vi "WLAN Configure Signal.vi"(0 "Instrument Handle In":refnum<k21>, 1 "Selector String":string, 5 "WLAN Signal Configuration":T1={"Auto Detect Signal?"=TRUE, "Standard"=0, "Channel Bandwidth (Hz)"=20000000.0} {"Channel Bandwidth (Hz)" items=["5M"=5000000.0, "10M"=10000000.0, "20M"=20000000.0, "40M"=40000000.0, "80M"=80000000.0, "160M"=160000000.0]; "Standard" items=["802.11a/g", "802.11b", "802.11j", "802.11p", "802.11n", "802.11ac", "802.11ax"]}, 11 "error in (no error)":errorcluster) -> (4 "Instrument Handle Out":refnum<k21>, 15 "error out":errorcluster)   [LabVIEW 2016, in "RFmxWLAN.lvlib"]
uses:
  RFmxWLAN.lvlib
  Typedefs/WLAN Signal Configuration.ctl
panel:
  # "OR"
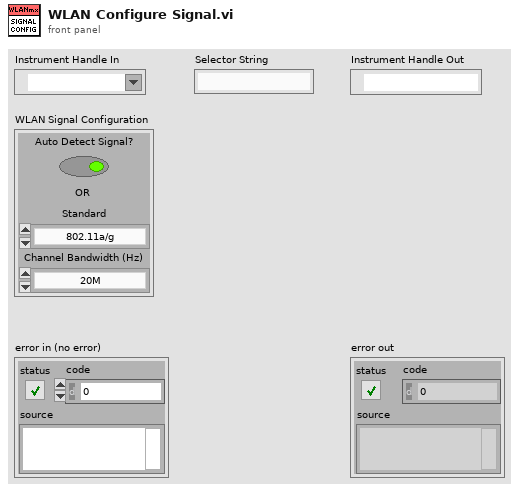
[diagram p1: front panel]
types:
  T1 = typedef "RFmxWLAN.lvlib/WLAN Signal Configuration.ctl" = cluster{"Auto Detect Signal?":bool, "Standard":i32, "Channel Bandwidth (Hz)":dbl}
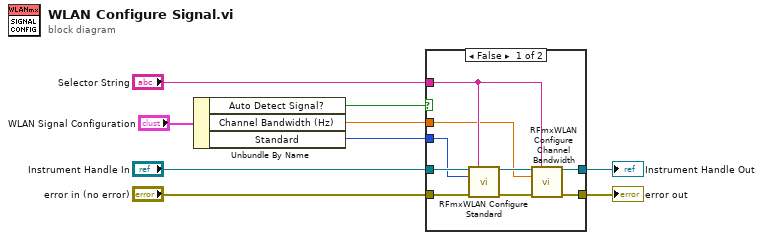
[diagram p0: block diagram]
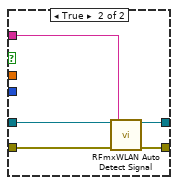
[diagram p2: hidden frame]
diagram:
  n1 = Unbundle By Name("WLAN Signal Configuration") -> ("Auto Detect Signal?"=w3:bool, "Channel Bandwidth (Hz)"=w2:dbl, "Standard"=w1:i32)
  n2 = case shown="False" w3 {
    tunnel: "Instrument Handle In" -> [w18 w23]
    tunnel: "error in (no error)" -> [w17 w22]
    tunnel: [w13 w21] -> w7
    tunnel: [w14 w20] -> w6
    tunnel: "Selector String" -> [w12 w19]
    tunnel: w2 -> [w11 _]
    tunnel: w1 -> [w10 _]
    frame False {
      n3 = call <vilib>:"RFmxWLAN Configure Standard.vi"("Instrument Handle In"=w18, "Selector String"=w12, "Standard"=w10, "error in (no error)"=w17) -> ("Instrument Handle Out"=w16:refnum<k21>, "error out"=w15:errorcluster)  [unwired: 10 in]
      n4 = call <vilib>:"RFmxWLAN Configure Channel Bandwidth.vi"("Instrument Handle In"=w16, "Selector String"=w12, "Channel Bandwidth (Hz)"=w11, "error in (no error)"=w15) -> ("Instrument Handle Out"=w14:refnum<k21>, "error out"=w13:errorcluster)  [unwired: 10 in]
    }
    frame True {
      n5 = call <vilib>:"RFmxWLAN Auto Detect Signal.vi"("Instrument Handle In"=w23, "Selector String"=w19, "error in (no error)"=w22) -> ("Instrument Handle Out"=w20:refnum<k21>, "error out"=w21:errorcluster)  [unwired: 11 in]
    }
  }
  "Instrument Handle Out" <- w6
  "error out" <- w7
